vi "save everything this project less crashy.vi"(8 "error in":errorcluster, 11 "Project in":refnum<vi>) -> (0 "error out":errorcluster, 3 "Project out":refnum<vi>)   [LabVIEW 2013, in "DCAFConfigurablePluginDecideFeatures.lvclass"]
doc: "Given a project reference, this VI saves all the VIs and libraries in the project and the project itself. This is equivalent to choosing the File >> Save All (This Project) menu item."
uses:
  DCAFConfigurablePluginDecideFeatures.lvclass
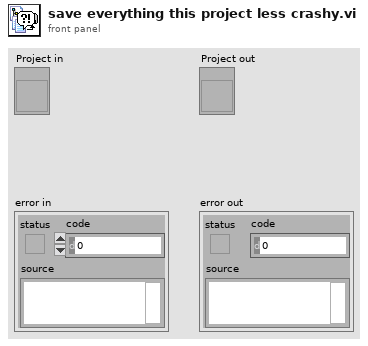
[diagram p1: front panel]
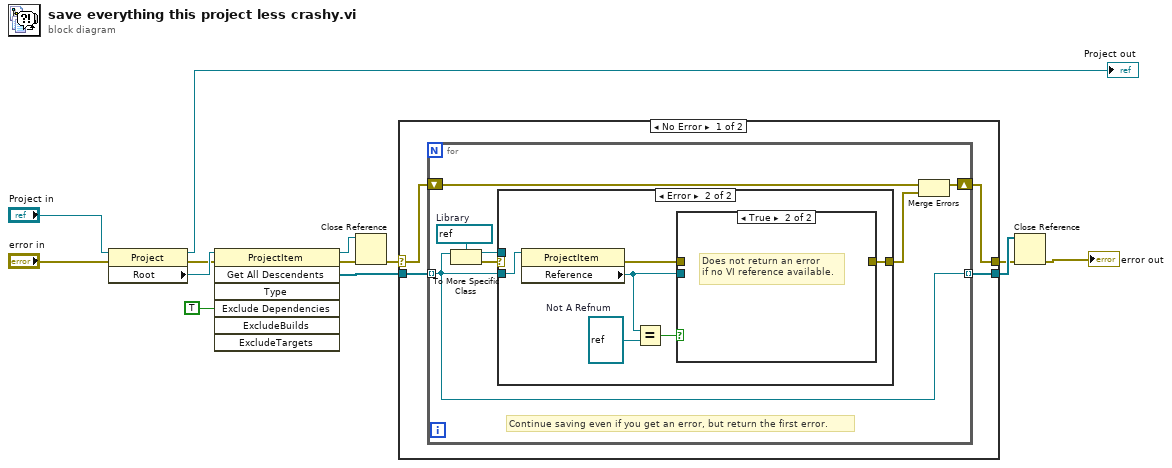
[diagram p0: block diagram]
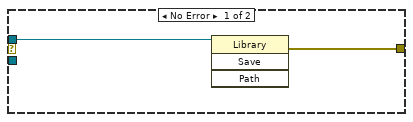
[diagram p2: hidden frame]
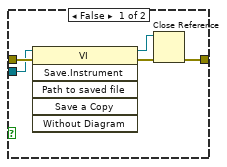
[diagram p3: hidden frame]
diagram:
  n1 = property class="Project"(reference="Project in", error in="error in") -> (reference out=→"Project out":refnum<vi>, error out=w2:errorcluster, "Root"=w8:refnum<vi>)
  n2 = invoke class="ProjectItem" method="Get All Descendents"(reference=w8, error in=w2, "Exclude Dependencies"=TRUE ("Exclude Dependencies? (F)")) -> (reference out=w10:refnum<vi>, error out=w11:errorcluster, "All Descendents"=w12:refnum<vi>[])  [unwired: 4 in, 4 out]
  n3 = Close Reference(reference=w10, error in (no error)=w11) -> (error out=w5:errorcluster)
  n4 = case shown="No Error" w5 {
    selector: w5 -> [w15 w39]
    tunnel: [w17 w38] -> w13
    tunnel: w12 -> [w16 w38]
    tunnel: [w14 w39] -> w4
    frame No Error {
      n5 = for {
        tunnel: w16 -> [w21] mode=indexing
        tunnel: [w21] -> w17 mode=indexing
        shift-right: [w19] -> w14
        shift-left: w15 -> [w20]
        w24 = refnum<vi> refnum  # Library
        # "Continue saving even if you get an error, but return the first error."
        n6 = To More Specific Class(target class=w24, reference=w21) -> (specific class reference=w23:refnum<vi>, error out=w22:errorcluster)  [unwired: 1 in]
        n7 = case shown="Error" w22 {
          tunnel: w23 -> [w26 _]
          tunnel: [w25 w27] -> w18
          tunnel: w21 -> [_ w31]
          frame No Error {
            n8 = invoke class="Library" method="Save"(reference=w26) -> (error out=w25:errorcluster)  [unwired: 3 in, 3 out]
          }
          frame Error {
            w30 = refnum<vi> refnum  # Not A Refnum
            n9 = property class="ProjectItem"(reference=w31) -> (error out=w32:errorcluster, "Reference"=w28:refnum<vi>)  [unwired: 1 in, 1 out]
            n10 = Equal?(x=w28, y=w30) -> (x = y?=w29:bool)
            n11 = case shown="True" w29 {
              tunnel: w32 -> [w37 _]
              tunnel: [w33 _] -> w27
              tunnel: w28 -> [w36 _]
              frame False {
                n12 = invoke class="VI" method="Save.Instrument"(reference=w36, error in=w37) -> (reference out=w35:refnum<vi>, error out=w34:errorcluster)  [unwired: 4 in, 4 out]
                n13 = Close Reference(reference=w35, error in (no error)=w34) -> (error out=w33:errorcluster)
              }
              frame True {
                # "Does not return an error\nif no VI reference available."
              }
            }
          }
        }
        n14 = Merge Errors(w20, w18) -> (w19:errorcluster)
      }
    }
    frame Error {
    }
  }
  n15 = Close Reference(reference=w13, error in (no error)=w4) -> (error out=→"error out":errorcluster)
